vi "LoadrefsFromFile.vi"(7 "error in":errorcluster, 9 "Numéro d'axe":i32, 10 "file path (use dialog)":path) -> (0 "error out":errorcluster, 2 "Références Chargées":i32[](array[numeric]))   [LabVIEW 2013]
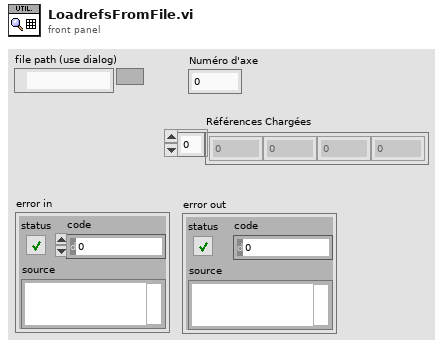
[diagram p1: front panel]
types:
  T1 = enum16{"open", "replace", "create", "open or create", "replace or create", "replace or create with confirmation"}
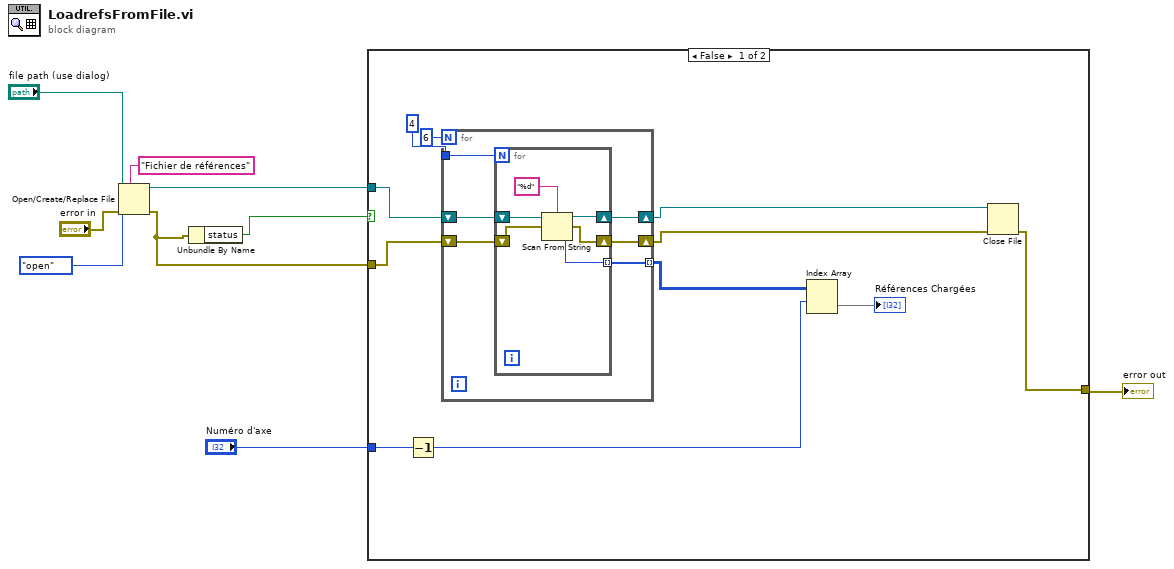
[diagram p0: block diagram]
diagram:
  n1 = Open/Create/Replace File(file path (use dialog)="file path (use dialog)", error in="error in", prompt="Fichier de références", operation (0:open)=T1."open") -> (refnum out=w7:refnum<file>, error out=w4:errorcluster)  [unwired: 2 in, 1 out]
  n2 = Unbundle By Name(w4) -> ("status"=w2:bool)
  n3 = case shown="False" w2 {
    tunnel: w4 -> [w17 w33]
    tunnel: w7 -> [w18 _]
    tunnel: [w20 w33] -> w6
    tunnel: "Numéro d'axe" -> [w13 _]
    frame False {
      n4 = Decrement(x=w13) -> (x-1=w11:i32)
      n5 = for {
        N: 6 -> [_]
        tunnel: 4 -> [w24]
        shift-right: [w22] -> w15
        shift-left: w17 -> [w25]
        shift-right: [w23] -> w16
        shift-left: w18 -> [w26]
        tunnel: [w21] -> w14 mode=indexing
        n6 = for {
          N: w24 -> [_]
          shift-right: [w29] -> w22
          shift-left: w25 -> [w31]
          shift-right: [w28] -> w23
          shift-left: w26 -> [w32]
          tunnel: [w27] -> w21 mode=indexing
          n7 = Scan From String("%d" ("format string"), w32, w31) -> (w28:refnum<file>, w29:errorcluster, output 1=w27:i32)  [unwired: 1 in]
        }
      }
      n8 = Index Array(array=w14, index (row)=w11) -> (element=→"Références Chargées":i32[])  [unwired: 1 in]
      n9 = Close File(refnum=w16, error in=w15) -> (error out=w20:errorcluster)  [unwired: 1 out]
    }
    frame True {
    }
  }
  "error out" <- w6
